vi "shift Scan Pattern.vi"(4 "error in (no error)":errorcluster, 5 "Shift Y":dbl, 6 "Shift X":dbl, 7 "Scan Pattern in":refnum<class "Scan Pattern.lvclass">) -> (0 "error out":errorcluster, 3 "Scan Pattern out":refnum<class "Scan Pattern.lvclass">)   [LabVIEW 2017]
uses:
  C:/Program Files/Thorlabs/SpectralRadar/LabVIEW/2012/user.lib/SpectralRadar.llb/Scan Pattern.lvclass
  SpectralRadar.dll
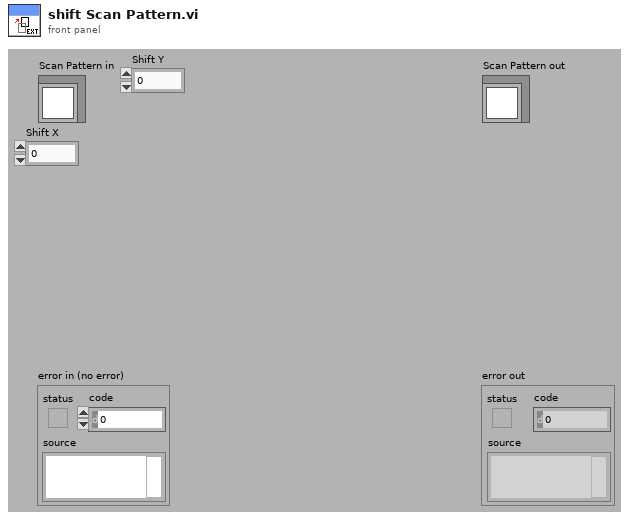
[diagram p1: front panel]
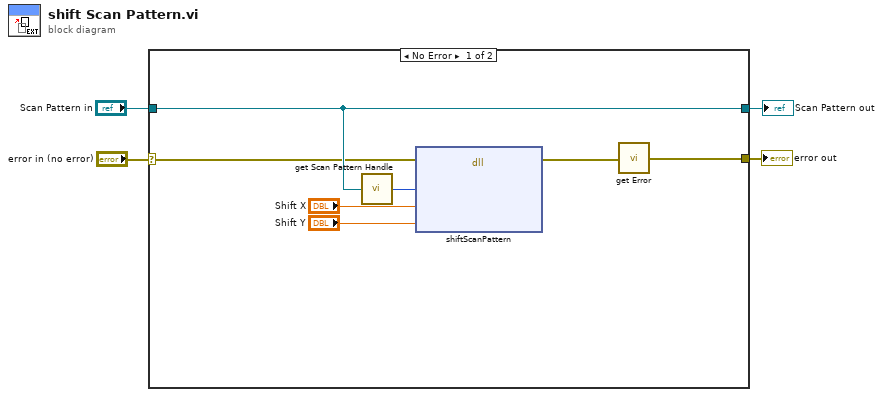
[diagram p0: block diagram]
diagram:
  n1 = case shown="No Error" "error in (no error)" {
    selector: "error in (no error)" -> [w10 w13]
    tunnel: [w5 w13] -> w3
    tunnel: [w11 w12] -> w1
    tunnel: "Scan Pattern in" -> [w11 w12]
    frame No Error {
      n2 = call "get Scan Pattern Handle.vi"("Scan Pattern"=w11) -> ("Handle"=w9:u64)
      n3 = dll-call lib="SpectralRadar.dll" fn="shiftScanPattern"(error in=w10, "Scan Pattern Handle"=w9, "Shift X"="Shift X", "Shift Y"="Shift Y") -> (error out=w6:errorcluster)  [unwired: 6 in, 1 out]
      n4 = call "get Error.vi"("error in (no error)"=w6) -> ("error out"=w5:errorcluster)
    }
    frame Error {
    }
  }
  "error out" <- w3
  "Scan Pattern out" <- w1
